vi "Write Data Directory.vi"(8 "error in (no error)":errorcluster, 10 "Data Directory":path, 11 "heater_parent in":refnum<class "heater_parent.lvclass">) -> (0 "error out":errorcluster, 3 "heater_parent out":refnum<class "heater_parent.lvclass">)   [LabVIEW 2020, in "polar_bear_plus_drivers.lvlib" / "heater_parent.lvclass"]
uses:
  <instrlib>/RxnRover/Driver Polar Bear Plus/heater_parent/heater_parent.lvclass
  <instrlib>/RxnRover/Driver Polar Bear Plus/heater_parent/heater_parent.lvclass/heater_parent.ctl
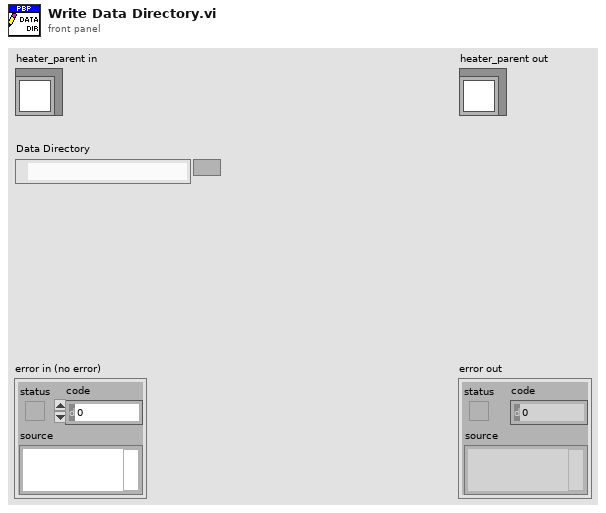
[diagram p1: front panel]
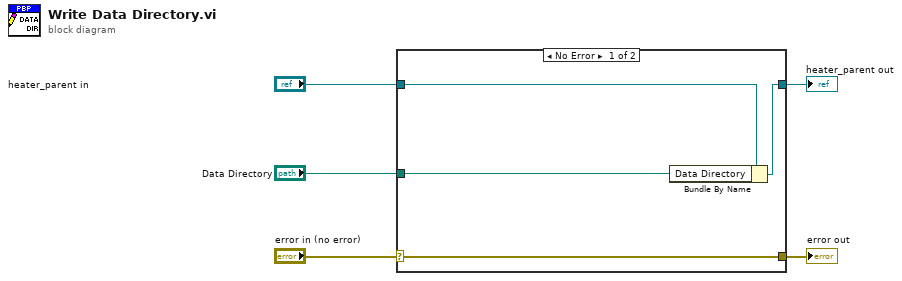
[diagram p0: block diagram]
diagram:
  n1 = case shown="No Error" "error in (no error)" {
    selector: "error in (no error)" -> [w9 w10]
    tunnel: [w9 w10] -> w4
    tunnel: [w7 w11] -> w2
    tunnel: "heater_parent in" -> [w8 w11]
    tunnel: "Data Directory" -> [w6 _]
    frame No Error {
      n2 = Bundle By Name(cluster=w8, "Data Directory"=w6) -> (w7:refnum<class "heater_parent.lvclass">)
    }
    frame Error {
    }
  }
  "error out" <- w4
  "heater_parent out" <- w2
